vi "GenerateAnalogWaveformPiezoTraj - FeedPiezoGalvo - GalvoPrecision.vi"(8 "error in (no error)":errorcluster, 11 "SetupInfo_IN":T1={"ConfigParameters_Analog"={"JAI camera fps"=240.0, "Bi-Lateral Galvo xy scan range (V)"=0.7, "Bi-Lateral Galvo xy scan frequency (Hz)"=500, "AOM Blind percent (%)"=0.1, "AOM start blind percent (%) "=70.0, "ROI threshold"=1.0, "AO Sampling rate"=1000000.0}, "ConfigParameters_Digital"={"Steps per volume"=25.0, "Time per volume (s)"=0.4, "OG start layer"=15.0, "Objective Lin Rising Vel (micron/ms）"=1.0, "Image depth (micron)"=200.0, "OG latency (s)"=10.0, "OG repitation"=3.0, "OG end layer"=17.0, "Shock1 duration (s)"=0.001, "Shock2 duration (s)"=0.001, "Shock3 duration (s)"=0.01, "Shock4 duration (s)"=0.01, "Shock5 duration (s)"=0.1, "Shock duration_New"=[]}, "ConfigParameters_Other1"={"Frontal Galvo xy scan range (V)"=0.14, "Frontal Galvo xy scan frequency (Hz)"=500, "PFI 0 digital clock frequency"=500000.0, "Window size for layer index"=0.5, "sCMOS fps"=95.0}, "ConfigParameters_Others2"={"#Trials baseline"=6, "#Trials test"=6, "Time before acq. (s)"=360.0, "Time before test (s)"=600.0, "#Blocks acquisition"=5, "Inter-trial interval baseline (s)"=60.0, "#Trials per acquition block"=6, "Inter-block interval acquisition (s)"=360.0, "Inter-trial interval acquisition (s)"=20.0, "Flash latency (s)"=10.0, "Flash duration (s)"=3.2, "Response duration (s)"=10.0, "MaxTimeEventDetection (s)"=6, "StimType"=enum."Flash", "#MaxEvents"=6}, "ProcessParametersOut"={"stand Z vol Acquisition time (s)"=0.2631578947368421, "stand Z vol Backward time (s)"=0.13684210526315793, "Objective scan volt"=5.0, "Bi-lateral Galvo Z scan volt"=0.1800000180000018, "Frontal Galvo Z scan volt"=0.14940000509752818, "Objective step length (micron)"=8.0, "OG Z volet Linear Dec time (s)"=0.024, "OG Z vol Stim. steps time (s)"=0.031578947368421054, "OG Z vol Linear Acc time (s)"=0.112, "#Vol. of flash"=8, "#Vol. of shock"=1, "#Vol. bef flash"=25, "#Vol. aft flash"=17, "OG Z vol Linear Dec time (s)"=0.112, "OG Z vol time (s)"=0.39073684210526316, "Stack duration"=[0.001, 0.001, 0.01, 0.01, 0.1], "AOM stand. value size"=400000, "Plane indexing length"=0, "#Vol. blank"=0, "#Vol. blank before acq"=0, "#Vol. blank before test"=0, " #Inter-block interval acquisition (Ed-St Vol)"=0}, "WaveformParameters"={"stand Z vol Acquisition samp info"={"Fs"=1000000.0, "#s"=263158.0}, "stand Z vol Backward samp info"={"Fs"=1000000.0, "#s"=136842.0}, "OG Z vol Linear Acc samp info"={"Fs"=1000000.0, "#s"=112000.0}, "OG Z vol Stim. steps samp info"={"Fs"=1000000.0, "#s"=31579.0}, "OG Z volet Linear Dec samp info"={"Fs"=1000000.0, "#s"=24000.0}, "OG Z vol Linear Dec samp info"={"Fs"=1000000.0, "#s"=112000.0}, "OG Z vol samp info"={"Fs"=1000000.0, "#s"=390737.0}, "stand Z vol backforth samp info"={"Fs"=1000000.0, "#s"=400000.0}}, "AnalogWaveform"={"Bi-lateral Galvo Z stand waveform"={"t0"=timestamp(0 s since 1904-01-01), "dt"=1.0, "Y"=[]}, "Frontal Galvo Z stand waveform"={"t0"=timestamp(0 s since 1904-01-01), "dt"=1.0, "Y"=[]}, "Bi-lateral Galvo XY stand waveform"={"t0"=timestamp(0 s since 1904-01-01), "dt"=1.0, "Y"=[]}, "Frontal Galvo XY stand waveform"={"t0"=timestamp(0 s since 1904-01-01), "dt"=1.0, "Y"=[]}, "sCMOS stand waveform"={"t0"=timestamp(0 s since 1904-01-01), "dt"=1.0, "Y"=[]}, "Detection objective stand waveform"={"t0"=timestamp(0 s since 1904-01-01), "dt"=1.0, "Y"=[]}, "AOM stand waveform"={"t0"=timestamp(0 s since 1904-01-01), "dt"=1.0, "Y"=[]}, "PFI 0 clock stand waveform"={"t0"=timestamp(0 s since 1904-01-01), "dt"=1.0, "Y"=[]}, "Bi-lateral Galvo Z OG waveform"={"t0"=timestamp(0 s since 1904-01-01), "dt"=1.0, "Y"=[]}, "Bi-lateral Galvo XY OG waveform"={"t0"=timestamp(0 s since 1904-01-01), "dt"=1.0, "Y"=[]}, "Frontal Galvo Z OG waveform"={"t0"=timestamp(0 s since 1904-01-01), "dt"=1.0, "Y"=[]}, "Frontal Galvo XY OG waveform"={"t0"=timestamp(0 s since 1904-01-01), "dt"=1.0, "Y"=[]}, "sCMOS OG waveform"={"t0"=timestamp(0 s since 1904-01-01), "dt"=1.0, "Y"=[]}, "Detection objective OG waveform"={"t0"=timestamp(0 s since 1904-01-01), "dt"=1.0, "Y"=[]}, "AOM OG waveform"={"t0"=timestamp(0 s since 1904-01-01), "dt"=1.0, "Y"=[]}, "PFI 0 clock OG wavee"={"t0"=timestamp(0 s since 1904-01-01), "dt"=1.0, "Y"=[]}, "sCMOS blank waveform"={"t0"=timestamp(0 s since 1904-01-01), "dt"=1.0, "Y"=[]}, "All analog OG wave"=[], "All analog stand wave"=[], "All analog blank wave"=[], "BufferWaveform_Analog"=[], "Bi-lateral Galvo Z XY"={"t0"=timestamp(0 s since 1904-01-01), "dt"=1.0, "Y"=[]}, "Frontal Galvo Z XY"={"t0"=timestamp(0 s since 1904-01-01), "dt"=1.0, "Y"=[]}, "sCMOS Trigger XY"={"t0"=timestamp(0 s since 1904-01-01), "dt"=1.0, "Y"=[]}, "Detection objective XY"={"t0"=timestamp(0 s since 1904-01-01), "dt"=1.0, "Y"=[]}, "AOM XY"={"t0"=timestamp(0 s since 1904-01-01), "dt"=1.0, "Y"=[]}, "Analog_XY"=[]}, "DigitalWaveform"={"AllDigitalStandWave"=[], "AllDigialEvokedWave"=[], "AllDigialOGWave"=[], "AllDigitalPairWave_1"=[], "AllDigitalPairWave_2"=[], "AllDigitalPairWave_3"=[], "AllDigitalPairWave_4"=[], "AllDigitalPairWave_5"=[], "Plane Indexing"={"t0"=timestamp(0 s since 1904-01-01), "dt"=0.0, "Y"={"transitions"=[], "data"=[]}, "error"={"status"=FALSE, "code"=37421928, "source"=""}}, "Plane indexing P0.5 OG"={"t0"=timestamp(0 s since 1904-01-01), "dt"=0.0, "Y"={"transitions"=[], "data"=[]}, "error"={"status"=FALSE, "code"=37421928, "source"=""}}, "AllDigitalPairWaves"=[], "BufferWaveform_Digital"=[], "AllDigitalBlankWave"=[], "Digial_XY"=[]}, "PhysicalResource"={"PhysicalChannels_AI"="", "PhysicalChannels_AO"="", "PhysicalChannels_DO"="", "Task_AnalogOutput"="", "Task_DigitalOutput"="", "Task_AnalogInput"=""}, "ControlsRef"={"Mode_1"=refnum, "EventDetectionMode"=refnum, "Mode_2A"=refnum, "StimulationMode"=refnum, "Mode_2B"=refnum, "ErrorMeg"=refnum}} {"ConfigParameters_Other1"."Frontal Galvo xy scan frequency (Hz)" min=500 max=500; "ConfigParameters_Other1"."Frontal Galvo xy scan range (V)" min=0.0 max=1.5; "ConfigParameters_Analog"."AOM start blind percent (%)" min=10.0 max=90.0; "ConfigParameters_Analog"."AOM Blind percent (%)" min=0.1 max=100.0; "ConfigParameters_Analog"."Bi-Lateral Galvo xy scan frequency (Hz)" min=500 max=500; "ConfigParameters_Analog"."Bi-Lateral Galvo xy scan range (V)" min=0.0 max=1.5}) -> (0 "error out":errorcluster, 3 "SetupInfo_OUT":T1={"ConfigParameters_Analog"={"JAI camera fps"=240.0, "Bi-Lateral Galvo xy scan range (V)"=0.7, "Bi-Lateral Galvo xy scan frequency (Hz)"=500, "AOM Blind percent (%)"=0.1, "AOM start blind percent (%) "=70.0, "ROI threshold"=1.0, "AO Sampling rate"=1000000.0}, "ConfigParameters_Digital"={"Steps per volume"=25.0, "Time per volume (s)"=0.4, "OG start layer"=15.0, "Objective Lin Rising Vel (micron/ms）"=1.0, "Image depth (micron)"=200.0, "OG latency (s)"=10.0, "OG repitation"=3.0, "OG end layer"=17.0, "Shock1 duration (s)"=0.001, "Shock2 duration (s)"=0.001, "Shock3 duration (s)"=0.01, "Shock4 duration (s)"=0.01, "Shock5 duration (s)"=0.1, "Shock duration_New"=[]}, "ConfigParameters_Other1"={"Frontal Galvo xy scan range (V)"=0.14, "Frontal Galvo xy scan frequency (Hz)"=500, "PFI 0 digital clock frequency"=500000.0, "Window size for layer index"=0.5, "sCMOS fps"=95.0}, "ConfigParameters_Others2"={"#Trials baseline"=6, "#Trials test"=6, "Time before acq. (s)"=360.0, "Time before test (s)"=600.0, "#Blocks acquisition"=5, "Inter-trial interval baseline (s)"=60.0, "#Trials per acquition block"=6, "Inter-block interval acquisition (s)"=360.0, "Inter-trial interval acquisition (s)"=20.0, "Flash latency (s)"=10.0, "Flash duration (s)"=3.2, "Response duration (s)"=10.0, "MaxTimeEventDetection (s)"=6, "StimType"=enum."Flash", "#MaxEvents"=6}, "ProcessParametersOut"={"stand Z vol Acquisition time (s)"=0.2631578947368421, "stand Z vol Backward time (s)"=0.13684210526315793, "Objective scan volt"=5.0, "Bi-lateral Galvo Z scan volt"=0.1800000180000018, "Frontal Galvo Z scan volt"=0.14940000509752818, "Objective step length (micron)"=8.0, "OG Z volet Linear Dec time (s)"=0.024, "OG Z vol Stim. steps time (s)"=0.031578947368421054, "OG Z vol Linear Acc time (s)"=0.112, "#Vol. of flash"=8, "#Vol. of shock"=1, "#Vol. bef flash"=25, "#Vol. aft flash"=17, "OG Z vol Linear Dec time (s)"=0.112, "OG Z vol time (s)"=0.39073684210526316, "Stack duration"=[0.001, 0.001, 0.01, 0.01, 0.1], "AOM stand. value size"=400000, "Plane indexing length"=0, "#Vol. blank"=0, "#Vol. blank before acq"=0, "#Vol. blank before test"=0, " #Inter-block interval acquisition (Ed-St Vol)"=0}, "WaveformParameters"={"stand Z vol Acquisition samp info"={"Fs"=1000000.0, "#s"=263158.0}, "stand Z vol Backward samp info"={"Fs"=1000000.0, "#s"=136842.0}, "OG Z vol Linear Acc samp info"={"Fs"=1000000.0, "#s"=112000.0}, "OG Z vol Stim. steps samp info"={"Fs"=1000000.0, "#s"=31579.0}, "OG Z volet Linear Dec samp info"={"Fs"=1000000.0, "#s"=24000.0}, "OG Z vol Linear Dec samp info"={"Fs"=1000000.0, "#s"=112000.0}, "OG Z vol samp info"={"Fs"=1000000.0, "#s"=390737.0}, "stand Z vol backforth samp info"={"Fs"=1000000.0, "#s"=400000.0}}, "AnalogWaveform"={"Bi-lateral Galvo Z stand waveform"={"t0"=timestamp(0 s since 1904-01-01), "dt"=1.0, "Y"=[]}, "Frontal Galvo Z stand waveform"={"t0"=timestamp(0 s since 1904-01-01), "dt"=1.0, "Y"=[]}, "Bi-lateral Galvo XY stand waveform"={"t0"=timestamp(0 s since 1904-01-01), "dt"=1.0, "Y"=[]}, "Frontal Galvo XY stand waveform"={"t0"=timestamp(0 s since 1904-01-01), "dt"=1.0, "Y"=[]}, "sCMOS stand waveform"={"t0"=timestamp(0 s since 1904-01-01), "dt"=1.0, "Y"=[]}, "Detection objective stand waveform"={"t0"=timestamp(0 s since 1904-01-01), "dt"=1.0, "Y"=[]}, "AOM stand waveform"={"t0"=timestamp(0 s since 1904-01-01), "dt"=1.0, "Y"=[]}, "PFI 0 clock stand waveform"={"t0"=timestamp(0 s since 1904-01-01), "dt"=1.0, "Y"=[]}, "Bi-lateral Galvo Z OG waveform"={"t0"=timestamp(0 s since 1904-01-01), "dt"=1.0, "Y"=[]}, "Bi-lateral Galvo XY OG waveform"={"t0"=timestamp(0 s since 1904-01-01), "dt"=1.0, "Y"=[]}, "Frontal Galvo Z OG waveform"={"t0"=timestamp(0 s since 1904-01-01), "dt"=1.0, "Y"=[]}, "Frontal Galvo XY OG waveform"={"t0"=timestamp(0 s since 1904-01-01), "dt"=1.0, "Y"=[]}, "sCMOS OG waveform"={"t0"=timestamp(0 s since 1904-01-01), "dt"=1.0, "Y"=[]}, "Detection objective OG waveform"={"t0"=timestamp(0 s since 1904-01-01), "dt"=1.0, "Y"=[]}, "AOM OG waveform"={"t0"=timestamp(0 s since 1904-01-01), "dt"=1.0, "Y"=[]}, "PFI 0 clock OG wavee"={"t0"=timestamp(0 s since 1904-01-01), "dt"=1.0, "Y"=[]}, "sCMOS blank waveform"={"t0"=timestamp(0 s since 1904-01-01), "dt"=1.0, "Y"=[]}, "All analog OG wave"=[], "All analog stand wave"=[], "All analog blank wave"=[], "BufferWaveform_Analog"=[], "Bi-lateral Galvo Z XY"={"t0"=timestamp(0 s since 1904-01-01), "dt"=1.0, "Y"=[]}, "Frontal Galvo Z XY"={"t0"=timestamp(0 s since 1904-01-01), "dt"=1.0, "Y"=[]}, "sCMOS Trigger XY"={"t0"=timestamp(0 s since 1904-01-01), "dt"=1.0, "Y"=[]}, "Detection objective XY"={"t0"=timestamp(0 s since 1904-01-01), "dt"=1.0, "Y"=[]}, "AOM XY"={"t0"=timestamp(0 s since 1904-01-01), "dt"=1.0, "Y"=[]}, "Analog_XY"=[]}, "DigitalWaveform"={"AllDigitalStandWave"=[], "AllDigialEvokedWave"=[], "AllDigialOGWave"=[], "AllDigitalPairWave_1"=[], "AllDigitalPairWave_2"=[], "AllDigitalPairWave_3"=[], "AllDigitalPairWave_4"=[], "AllDigitalPairWave_5"=[], "Plane Indexing"={"t0"=timestamp(0 s since 1904-01-01), "dt"=0.0, "Y"={"transitions"=[], "data"=[]}, "error"={"status"=FALSE, "code"=37421928, "source"=""}}, "Plane indexing P0.5 OG"={"t0"=timestamp(0 s since 1904-01-01), "dt"=0.0, "Y"={"transitions"=[], "data"=[]}, "error"={"status"=FALSE, "code"=37421928, "source"=""}}, "AllDigitalPairWaves"=[], "BufferWaveform_Digital"=[], "AllDigitalBlankWave"=[], "Digial_XY"=[]}, "PhysicalResource"={"PhysicalChannels_AI"="", "PhysicalChannels_AO"="", "PhysicalChannels_DO"="", "Task_AnalogOutput"="", "Task_DigitalOutput"="", "Task_AnalogInput"=""}, "ControlsRef"={"Mode_1"=refnum, "EventDetectionMode"=refnum, "Mode_2A"=refnum, "StimulationMode"=refnum, "Mode_2B"=refnum, "ErrorMeg"=refnum}} {"ConfigParameters_Other1"."Frontal Galvo xy scan frequency (Hz)" min=500 max=500; "ConfigParameters_Other1"."Frontal Galvo xy scan range (V)" min=0.0 max=1.5; "ConfigParameters_Analog"."AOM start blind percent (%)" min=10.0 max=90.0; "ConfigParameters_Analog"."AOM Blind percent (%)" min=0.1 max=100.0; "ConfigParameters_Analog"."Bi-Lateral Galvo xy scan frequency (Hz)" min=500 max=500; "ConfigParameters_Analog"."Bi-Lateral Galvo xy scan range (V)" min=0.0 max=1.5})   [LabVIEW 2018]
uses:
  SetupInfo.ctl
  ConfigParameters_Analog.ctl
  ConfigParameters_Digital.ctl
  ConfigParameters_Others1.ctl
  ConfigParameters_Others2.ctl
  ProcessParametersOut.ctl
  WaveformParameters.ctl
  AnalogWaveform.ctl
  DigitalWaveform.ctl
  PhysicalResource.ctl
  ControlsRef.ctl
  <vilib>/Waveform/WDTOps.llb/WDT Append Waveforms DBL.vi
  <vilib>/measure/NI_MABase.lvlib
panel:
  out "x/y":waveform(dbl)(graph)
  in  "FileSamplingRate":dbl=1000.0
  in  "PiezoTrajectoryPath":path=path "D:/APP/LightSheetController_Ver8 obl/VISource/Waveform/piezo_In_Out.txt"
  out "AOM stand. value size":i32=400000
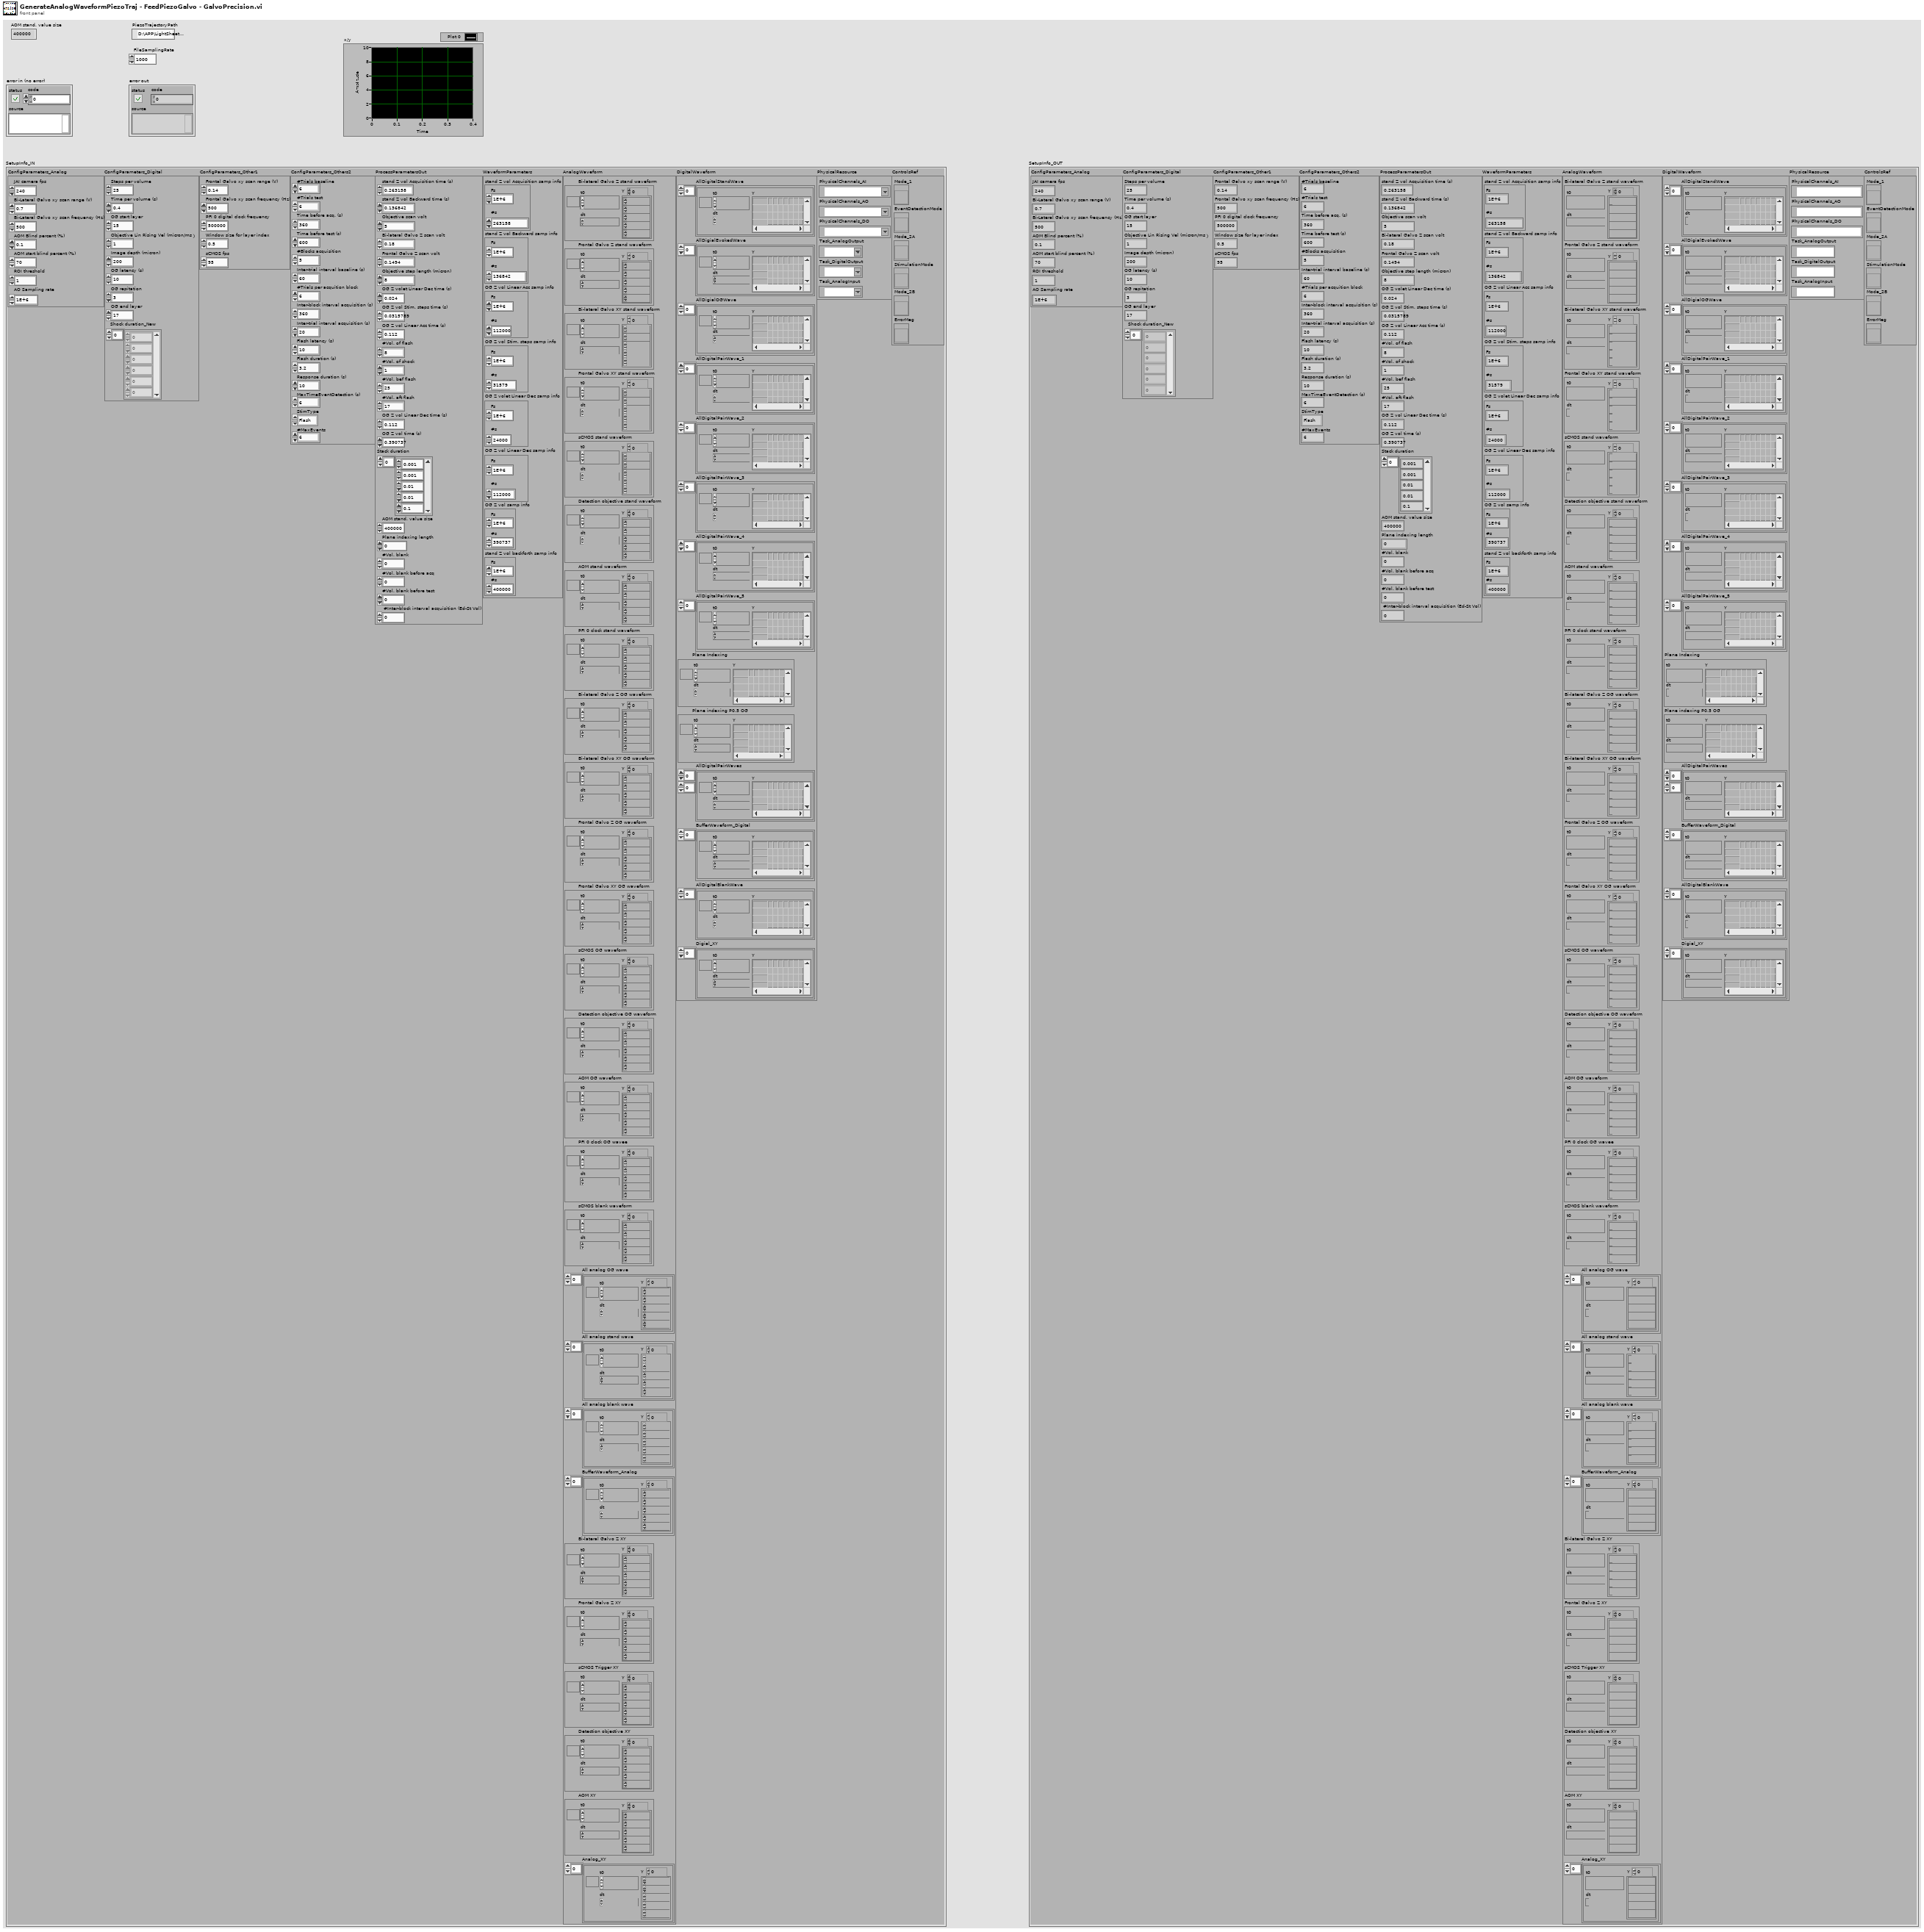
[diagram p1: front panel]
types:
  T1 = typedef "SetupInfo.ctl" = cluster{"ConfigParameters_Analog":T2, "ConfigParameters_Digital":T3, "ConfigParameters_Other1":T4, "ConfigParameters_Others2":T5, "ProcessParametersOut":T6, "WaveformParameters":T7, "AnalogWaveform":T8, "DigitalWaveform":T9, "PhysicalResource":T10, "ControlsRef":T11}
  T2 = typedef "ConfigParameters_Analog.ctl" = cluster{"JAI camera fps":dbl, "Bi-Lateral Galvo xy scan range (V)":dbl, "Bi-Lateral Galvo xy scan frequency (Hz)":i16, "AOM Blind percent (%)":dbl, "AOM start blind percent (%) ":dbl, "ROI threshold":dbl, "AO Sampling rate":dbl}
  T3 = typedef "ConfigParameters_Digital.ctl" = cluster{"Steps per volume":dbl, "Time per volume (s)":dbl, "OG start layer":dbl, "Objective Lin Rising Vel (micron/ms）":dbl, "Image depth (micron)":dbl, "OG latency (s)":dbl, "OG repitation":dbl, "OG end layer":dbl, "Shock1 duration (s)":dbl, "Shock2 duration (s)":dbl, "Shock3 duration (s)":dbl, "Shock4 duration (s)":dbl, "Shock5 duration (s)":dbl, "Shock duration_New":dbl[]}
  T4 = typedef "ConfigParameters_Others1.ctl" = cluster{"Frontal Galvo xy scan range (V)":dbl, "Frontal Galvo xy scan frequency (Hz)":i16, "PFI 0 digital clock frequency":dbl, "Window size for layer index":dbl, "sCMOS fps":dbl}
  T5 = typedef "ConfigParameters_Others2.ctl" = cluster{"#Trials baseline":i32, "#Trials test":i32, "Time before acq. (s)":dbl, "Time before test (s)":dbl, "#Blocks acquisition":i32, "Inter-trial interval baseline (s)":dbl, "#Trials per acquition block":i32, "Inter-block interval acquisition (s)":dbl, "Inter-trial interval acquisition (s)":dbl, "Flash latency (s)":dbl, "Flash duration (s)":dbl, "Response duration (s)":dbl, "MaxTimeEventDetection (s)":i32, "StimType":enum16{"Flash", "OG"}, "#MaxEvents":i32}
  T6 = typedef "ProcessParametersOut.ctl" = cluster{"stand Z vol Acquisition time (s)":dbl, "stand Z vol Backward time (s)":dbl, "Objective scan volt":dbl, "Bi-lateral Galvo Z scan volt":dbl, "Frontal Galvo Z scan volt":dbl, "Objective step length (micron)":dbl, "OG Z volet Linear Dec time (s)":dbl, "OG Z vol Stim. steps time (s)":dbl, "OG Z vol Linear Acc time (s)":dbl, "#Vol. of flash":i32, "#Vol. of shock":i32, "#Vol. bef flash":i32, "#Vol. aft flash":i32, "OG Z vol Linear Dec time (s)":dbl, "OG Z vol time (s)":dbl, "Stack duration":dbl[], "AOM stand. value size":i32, "Plane indexing length":i32, "#Vol. blank":i32, "#Vol. blank before acq":i32, "#Vol. blank before test":i32, " #Inter-block interval acquisition (Ed-St Vol)":i32}
  T7 = typedef "WaveformParameters.ctl" = cluster{"stand Z vol Acquisition samp info":cluster{"Fs":dbl, "#s":dbl}, "stand Z vol Backward samp info":cluster{"Fs":dbl, "#s":dbl}, "OG Z vol Linear Acc samp info":cluster{"Fs":dbl, "#s":dbl}, "OG Z vol Stim. steps samp info":cluster{"Fs":dbl, "#s":dbl}, "OG Z volet Linear Dec samp info":cluster{"Fs":dbl, "#s":dbl}, "OG Z vol Linear Dec samp info":cluster{"Fs":dbl, "#s":dbl}, "OG Z vol samp info":cluster{"Fs":dbl, "#s":dbl}, "stand Z vol backforth samp info":cluster{"Fs":dbl, "#s":dbl}}
  T8 = typedef "AnalogWaveform.ctl" = cluster{"Bi-lateral Galvo Z stand waveform":waveform(dbl), "Frontal Galvo Z stand waveform":waveform(dbl), "Bi-lateral Galvo XY stand waveform":waveform(dbl), "Frontal Galvo XY stand waveform":waveform(dbl), "sCMOS stand waveform":waveform(dbl), "Detection objective stand waveform":waveform(dbl), "AOM stand waveform":waveform(dbl), "PFI 0 clock stand waveform":waveform(dbl), "Bi-lateral Galvo Z OG waveform":waveform(dbl), "Bi-lateral Galvo XY OG waveform":waveform(dbl), "Frontal Galvo Z OG waveform":waveform(dbl), "Frontal Galvo XY OG waveform":waveform(dbl), "sCMOS OG waveform":waveform(dbl), "Detection objective OG waveform":waveform(dbl), "AOM OG waveform":waveform(dbl), "PFI 0 clock OG wavee":waveform(dbl), "sCMOS blank waveform":waveform(dbl), "All analog OG wave":waveform(dbl)[], "All analog stand wave":waveform(dbl)[], "All analog blank wave":waveform(dbl)[], "BufferWaveform_Analog":waveform(dbl)[], "Bi-lateral Galvo Z XY":waveform(dbl), "Frontal Galvo Z XY":waveform(dbl), "sCMOS Trigger XY":waveform(dbl), "Detection objective XY":waveform(dbl), "AOM XY":waveform(dbl), "Analog_XY":waveform(dbl)[]}
  T9 = typedef "DigitalWaveform.ctl" = cluster{"AllDigitalStandWave":digitalwaveform[], "AllDigialEvokedWave":digitalwaveform[], "AllDigialOGWave":digitalwaveform[], "AllDigitalPairWave_1":digitalwaveform[], "AllDigitalPairWave_2":digitalwaveform[], "AllDigitalPairWave_3":digitalwaveform[], "AllDigitalPairWave_4":digitalwaveform[], "AllDigitalPairWave_5":digitalwaveform[], "Plane Indexing":digitalwaveform, "Plane indexing P0.5 OG":digitalwaveform, "AllDigitalPairWaves":digitalwaveform[][], "BufferWaveform_Digital":digitalwaveform[], "AllDigitalBlankWave":digitalwaveform[], "Digial_XY":digitalwaveform[]}
  T10 = typedef "PhysicalResource.ctl" = cluster{"PhysicalChannels_AI":tag, "PhysicalChannels_AO":tag, "PhysicalChannels_DO":tag, "Task_AnalogOutput":refnum<k21>, "Task_DigitalOutput":refnum<k21>, "Task_AnalogInput":refnum<k21>}
  T11 = typedef "ControlsRef.ctl" = cluster{"Mode_1":refnum<vi>, "EventDetectionMode":refnum<vi>, "Mode_2A":refnum<vi>, "StimulationMode":refnum<vi>, "Mode_2B":refnum<vi>, "ErrorMeg":refnum<vi>}
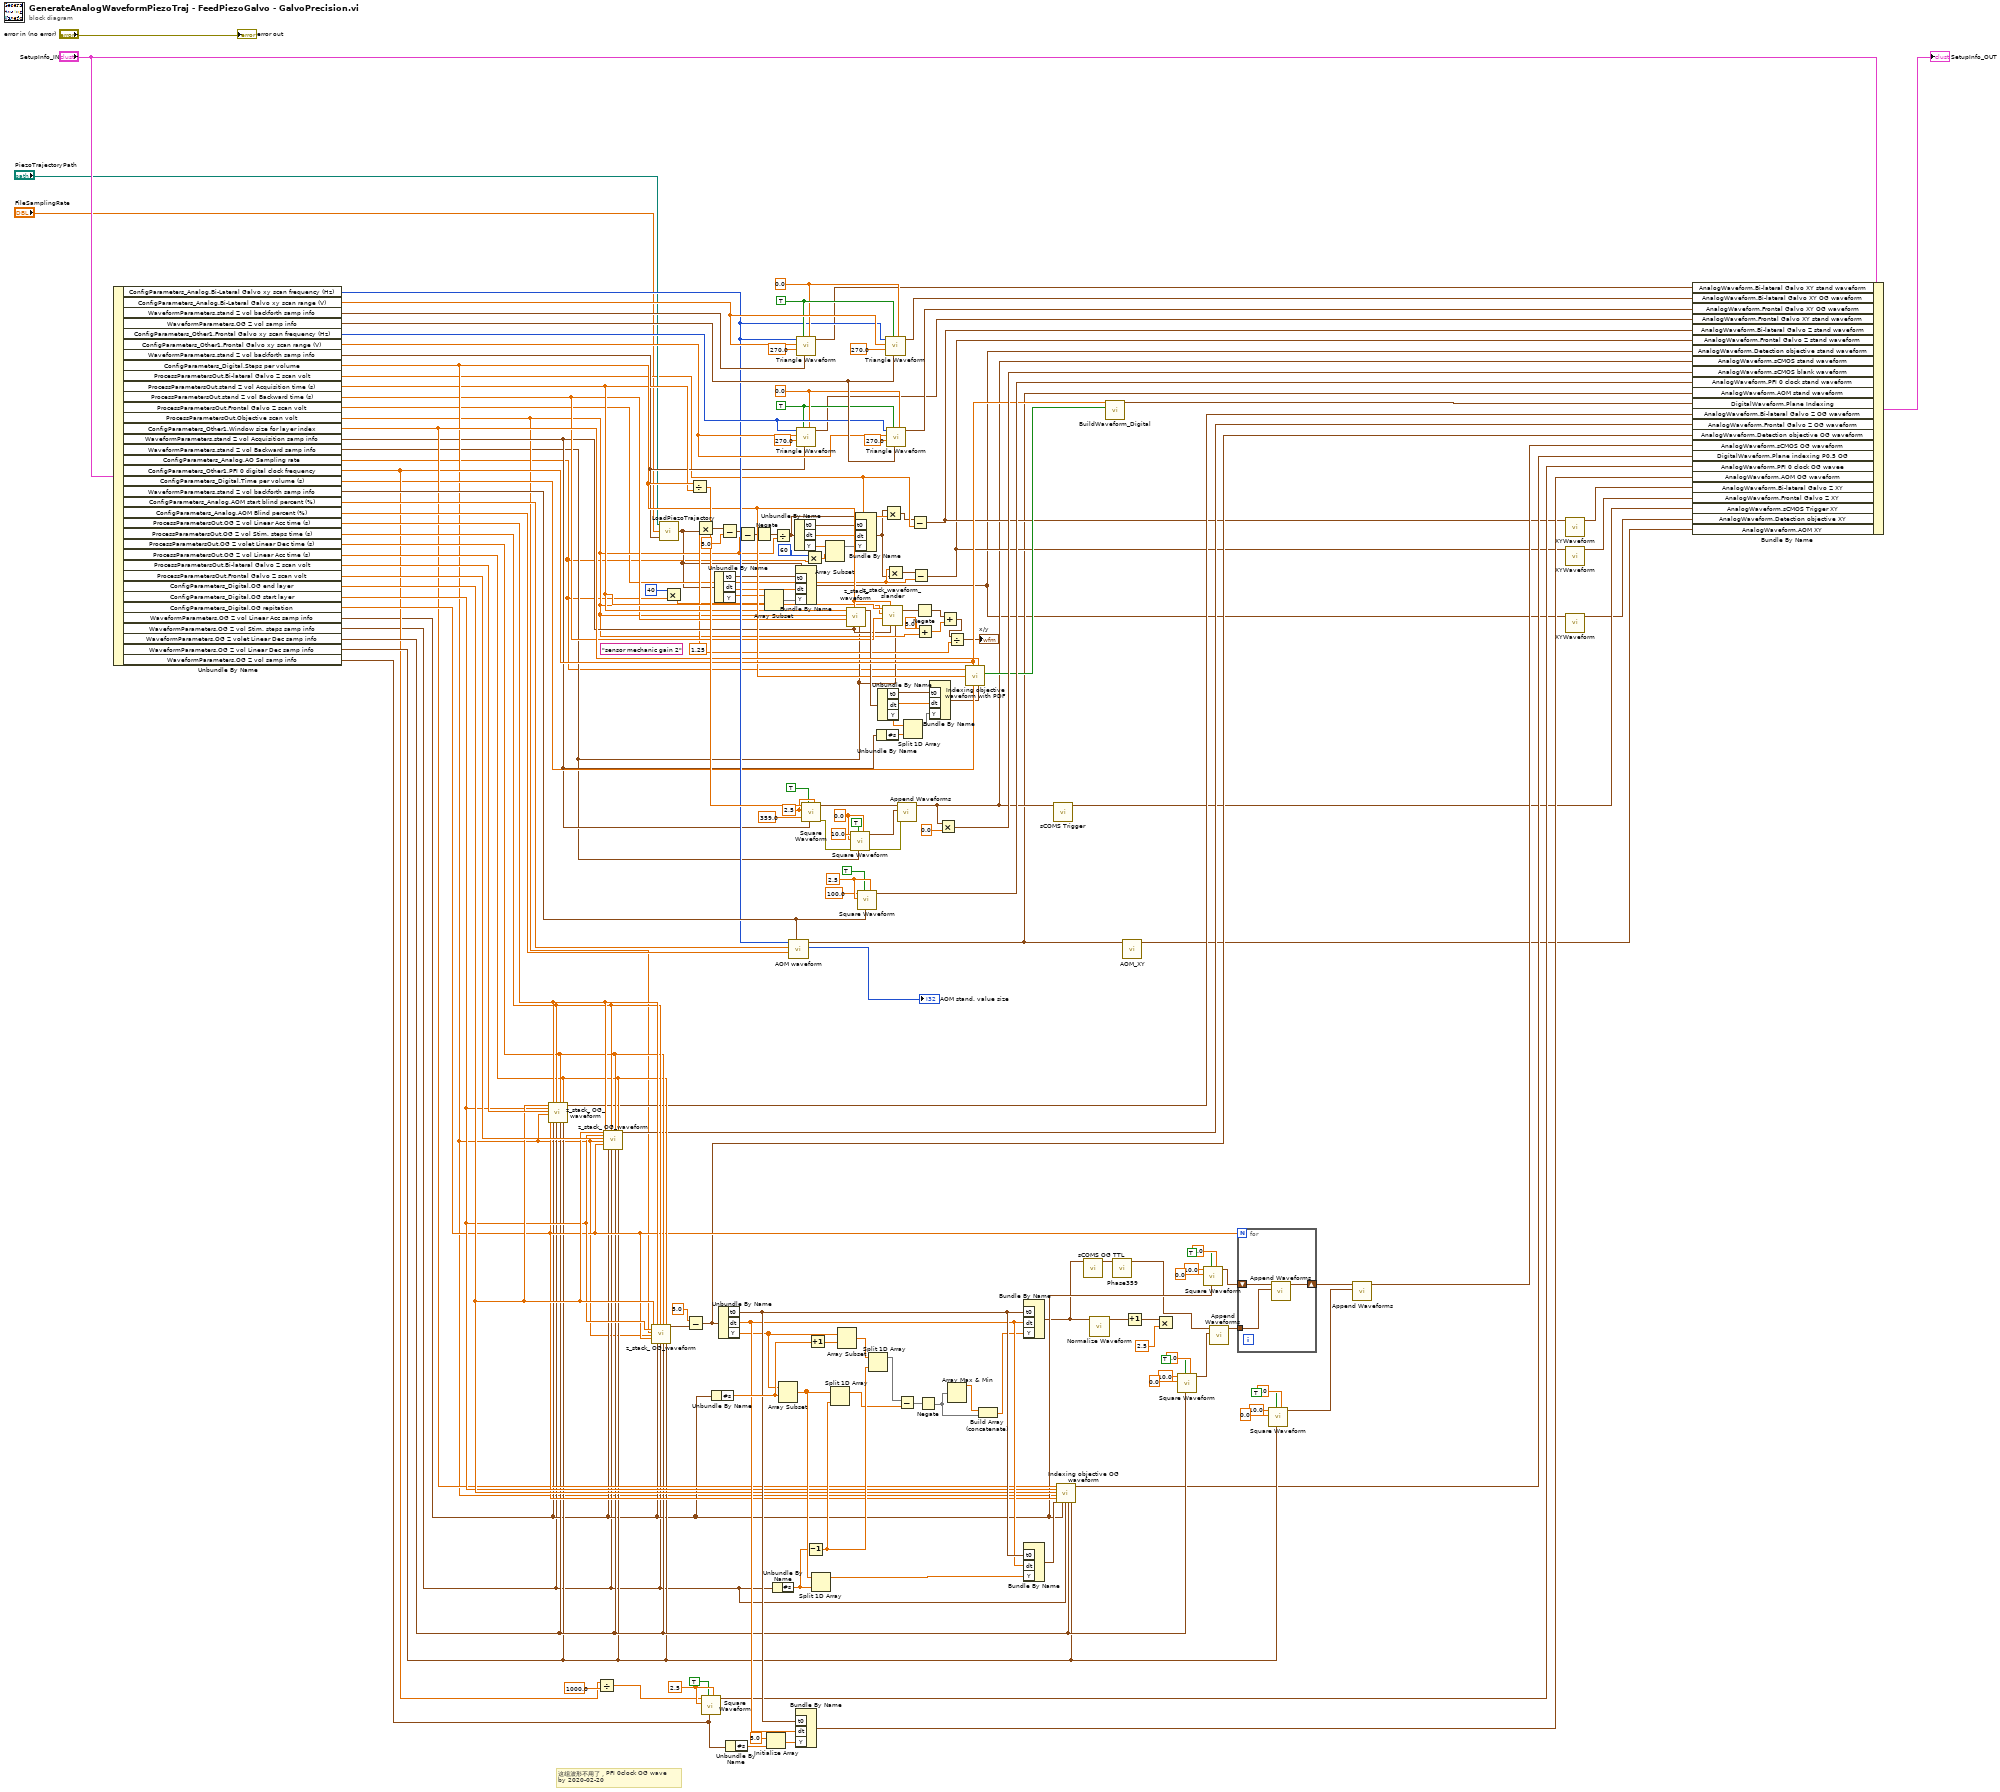
[diagram p0: block diagram]
diagram:
  (unwired) "sensor mechanic gain 2"
  w32 = 1.25
  w106 = 2.5
  w150 = 2.5 ("offset")
  w157 = 0.0 ("offset")
  w161 = 2.5 ("amplitude")
  w136 = TRUE ("reset signal")
  w144 = TRUE ("reset signal")
  w143 = 0.0 ("offset")
  w137 = 0.0 ("offset")
  # "这组波形不用了，PFI 0clock OG wave\nby 2020-02-20"
  n1 = Unbundle By Name("SetupInfo_IN") -> ("ConfigParameters_Analog.Bi-Lateral Galvo xy scan frequency (Hz)"=w133:i16, "ConfigParameters_Analog.Bi-Lateral Galvo xy scan range (V)"=w146:dbl, "WaveformParameters.stand Z vol backforth samp info"=w145:cluster{"Fs":dbl, "#s":dbl}, "WaveformParameters.OG Z vol samp info"=w141:cluster{"Fs":dbl, "#s":dbl}, "ConfigParameters_Other1.Frontal Galvo xy scan frequency (Hz)"=w140:i16, "ConfigParameters_Other1.Frontal Galvo xy scan range (V)"=w139:dbl, "WaveformParameters.stand Z vol backforth samp info"=w34:cluster{"Fs":dbl, "#s":dbl}, "ConfigParameters_Digital.Steps per volume"=w39:dbl, "ProcessParametersOut.Bi-lateral Galvo Z scan volt"=w24:dbl, "ProcessParametersOut.stand Z vol Acquisition time (s)"=w38:dbl, "ProcessParametersOut.stand Z vol Backward time (s)"=w37:dbl, "ProcessParametersOut.Frontal Galvo Z scan volt"=w22:dbl, "ProcessParametersOut.Objective scan volt"=w25:dbl, "ConfigParameters_Other1.Window size for layer index"=w90:dbl, "WaveformParameters.stand Z vol Acquisition samp info"=w36:cluster{"Fs":dbl, "#s":dbl}, "WaveformParameters.stand Z vol Backward samp info"=w20:cluster{"Fs":dbl, "#s":dbl}, "ConfigParameters_Analog.AO Sampling rate"=w3:dbl, "ConfigParameters_Other1.PFI 0 digital clock frequency"=w74:dbl, "ConfigParameters_Digital.Time per volume (s)"=w73:dbl, "WaveformParameters.stand Z vol backforth samp info"=w134:cluster{"Fs":dbl, "#s":dbl}, "ConfigParameters_Analog.AOM start blind percent (%)"=w132:dbl, "ConfigParameters_Analog.AOM Blind percent (%)"=w131:dbl, "ProcessParametersOut.OG Z vol Linear Acc time (s)"=w99:dbl, "ProcessParametersOut.OG Z vol Stim. steps time (s)"=w98:dbl, "ProcessParametersOut.OG Z volet Linear Dec time (s)"=w97:dbl, "ProcessParametersOut.OG Z vol Linear Acc time (s)"=w96:dbl, "ProcessParametersOut.Bi-lateral Galvo Z scan volt"=w95:dbl, "ProcessParametersOut.Frontal Galvo Z scan volt"=w94:dbl, "ConfigParameters_Digital.OG end layer"=w93:dbl, "ConfigParameters_Digital.OG start layer"=w92:dbl, "ConfigParameters_Digital.OG repitation"=w91:dbl, "WaveformParameters.OG Z vol Linear Acc samp info"=w56:cluster{"Fs":dbl, "#s":dbl}, "WaveformParameters.OG Z vol Stim. steps samp info"=w55:cluster{"Fs":dbl, "#s":dbl}, "WaveformParameters.OG Z volet Linear Dec samp info"=w89:cluster{"Fs":dbl, "#s":dbl}, "WaveformParameters.OG Z vol Linear Dec samp info"=w88:cluster{"Fs":dbl, "#s":dbl}, "WaveformParameters.OG Z vol samp info"=w87:cluster{"Fs":dbl, "#s":dbl})
  n2 = call "z_stack_ OG_waveform.vi"("OG end layer"=w93, "OG start layer"=w92, "SPECIFIC scan volt"=w95, "Steps per volume"=w39, "OG repitation"=w91, "Objective线性加速时间"=w99, "OG Z stack 线性加速 采样信息"=w56, "Objective 刺激steps 时间（s）"=w98, "OG Z stack 刺激steps 采样信息"=w55, "Objective volet 线性减速 时间（s）"=w97, "OG Z volet 线性减速 采样信息"=w89, "Objective线性减速时间"=w96, "OG Z stack 线性减速 采样信息"=w88) -> ("waveform out"=w77:waveform(dbl))  [unwired: 2 in, 4 out]
  n3 = Divide(x=w74, y=1000.0) -> (x/y=w80:dbl)
  n4 = call "z_stack_ OG_waveform.vi"("OG end layer"=w93, "OG start layer"=w92, "SPECIFIC scan volt"=w94, "Steps per volume"=w39, "OG repitation"=w91, "Objective线性加速时间"=w99, "OG Z stack 线性加速 采样信息"=w56, "Objective 刺激steps 时间（s）"=w98, "OG Z stack 刺激steps 采样信息"=w55, "Objective volet 线性减速 时间（s）"=w97, "OG Z volet 线性减速 采样信息"=w89, "Objective线性减速时间"=w96, "OG Z stack 线性减速 采样信息"=w88) -> ("waveform out"=w76:waveform(dbl))  [unwired: 2 in, 4 out]
  n5 = call "z_stack_ OG_waveform.vi"("OG end layer"=w93, "OG start layer"=w92, "SPECIFIC scan volt"=w25, "Steps per volume"=w39, "OG repitation"=w91, "Objective线性加速时间"=w99, "OG Z stack 线性加速 采样信息"=w56, "Objective 刺激steps 时间（s）"=w98, "OG Z stack 刺激steps 采样信息"=w55, "Objective volet 线性减速 时间（s）"=w97, "OG Z volet 线性减速 采样信息"=w89, "Objective线性减速时间"=w96, "OG Z stack 线性减速 采样信息"=w88) -> ("waveform out"=w69:waveform(dbl))  [unwired: 2 in, 4 out]
  n6 = call "LoadPiezoTrajactory.vi"("Z backforth 采样信息"=w34, "File Sampling Rate"="FileSamplingRate", "Path"="PiezoTrajectoryPath") -> ("output waveform"=w8:waveform(dbl))
  n7 = Multiply(x=40, y=w3) -> (x*y=w5:dbl)
  n8 = Subtract(x=5.0, y=w69) -> (x-y=w64:waveform(dbl))
  n9 = Divide(x=w39, y=w38) -> (x/y=w162:dbl)
  n10 = Multiply(x=w32, y=w8) -> (x*y=w31:waveform(dbl))
  n11 = call <vilib>:"Square Waveform.vi"("offset"=w106, "sampling info"=w87, "reset signal"=TRUE, "amplitude"=w106, "frequency"=w80) -> ("signal out"=w85:waveform(dbl))  [unwired: 5 in, 1 out]
  n12 = Unbundle By Name(w56) -> ("#s"=w107:dbl)
  n13 = Unbundle By Name(w8) -> ("t0"=w10:timestamp, "dt"=w9:dbl, "Y"=w6:dbl[])
  n14 = Unbundle By Name(w64) -> ("t0"=w102:timestamp, "dt"=w101:dbl, "Y"=w67:dbl[])
  n15 = Subtract(x=w31, y=5.0) -> (x-y=w30:waveform(dbl))
  n16 = Unbundle By Name(w87) -> ("#s"=w100:dbl)
  n17 = Subtract(x=w30, y=w25) -> (x-y=w27:waveform(dbl))
  n18 = Negate(x=w27) -> (-x=w26:waveform(dbl))
  n19 = Array Subset(array=w6, index=w5) -> (w7:dbl[])  [unwired: 1 in]
  n20 = Initialize Array(5.0 ("element"), w100) -> (w103:dbl[])
  n21 = Unbundle By Name(w55) -> ("#s"=w108:dbl)
  n22 = Divide(x=w26, y=w25) -> (x/y=w13:waveform(dbl))
  n23 = Array Subset(array=w67, index=w107) -> (w124:dbl[])  [unwired: 1 in]
  n24 = call "AOM waveform.vi"("z stack 往复采样信息"=w134, "AOM Blind percent (%)"=w131, "AOM start blind percent (%)"=w132, "Bi-Lateral Galvo xy scan frequency (Hz)"=w133) -> ("数值"=→"AOM stand. value size":i32, "Waveform"=w41:waveform(dbl))  [unwired: 6 in]
  n25 = Unbundle By Name(w13) -> ("t0"=w14:timestamp, "dt"=w17:dbl, "Y"=w15:dbl[])
  n26 = Bundle By Name(cluster=w8, "t0"=w10, "dt"=w9, "Y"=w7) -> (w11:waveform(dbl))
  n27 = Bundle By Name("t0"=w102, "dt"=w101, "Y"=w103) -> (w84:waveform(dbl))  [unwired: 1 in]
  n28 = call <vilib>:"Triangle Waveform.vi"("offset"=w143, "sampling info"=w145, "reset signal"=w144, "phase"=270.0, "amplitude"=w146, "frequency"=w133) -> ("signal out"=w82:waveform(dbl))  [unwired: 4 in, 1 out]
  n29 = call <vilib>:"Triangle Waveform.vi"("offset"=w137, "sampling info"=w34, "reset signal"=w136, "phase"=270.0, "amplitude"=w139, "frequency"=w140) -> ("signal out"=w135:waveform(dbl))  [unwired: 4 in, 1 out]
  n30 = call <vilib>:"Square Waveform.vi"("offset"=w161, "sampling info"=w36, "reset signal"=TRUE, "phase"=359.0, "amplitude"=w161, "frequency"=w162) -> ("error out"=w155:errorcluster, "signal out"=w153:waveform(dbl))  [unwired: 4 in]
  n31 = Multiply(x=60, y=w3) -> (x*y=w4:dbl)
  n32 = Decrement(x=w108) -> (x-1=w125:dbl)
  n33 = Increment(x=w107) -> (x+1=w126:dbl)
  n34 = Split 1D Array(array=w124, index=w108) -> (first subarray=w123:dbl[])  [unwired: 1 out]
  n35 = Array Subset(array=w15, index=w4) -> (w12:dbl[])  [unwired: 1 in]
  n36 = Split 1D Array(array=w124, index=w125) -> (first subarray=w60:dbl[])  [unwired: 1 out]
  n37 = Array Subset(array=w67, index=w126) -> (w66:dbl[])  [unwired: 1 in]
  n38 = call "z_stack_waveform.vi"("Z stack backward"=w20, "Z stack acquisition"=w36, "Steps per Volume"=w39, "Backward Time (s)"=w37, "SPECIFIC scan volt"=w25, "Aquisition Time (s)"=w38) -> ("WaveformOut"=w71:waveform(dbl))  [unwired: 5 in]
  n39 = call <vilib>:"Square Waveform.vi"("offset"=w157, "sampling info"=w20, "reset signal"=TRUE, "error in (no error)"=w155, "amplitude"=w157, "frequency"=10.0) -> ("error out"=w152:errorcluster, "signal out"=w154:waveform(dbl))  [unwired: 4 in]
  n40 = Bundle By Name(cluster=w13, "t0"=w14, "dt"=w17, "Y"=w12) -> (w16:waveform(dbl))
  n41 = call <vilib>:"Square Waveform.vi"("offset"=w150, "sampling info"=w134, "reset signal"=TRUE, "amplitude"=w150, "frequency"=100.0 ("amplitude")) -> ("signal out"=w129:waveform(dbl))  [unwired: 5 in, 1 out]
  n42 = Split 1D Array(array=w66, index=w125) -> (first subarray=w61:dbl[])  [unwired: 1 out]
  n43 = Unbundle By Name(w36) -> ("#s"=w164:dbl)
  n44 = Unbundle By Name(w71) -> ("t0"=w167:timestamp, "dt"=w166:dbl, "Y"=w165:dbl[])
  n45 = call "z_stack_waveform_slander.vi"("Z stack backward"=w20, "Z stack acquisition"=w36, "Steps per Volume"=w39, "Backward Time (s)"=w37, "SPECIFIC scan volt"=w25, "Aquisition Time (s)"=w38) -> ("WaveformOut"=w40:waveform(dbl))  [unwired: 5 in]
  n46 = Multiply(x=w16, y=w24) -> (x*y=w23:waveform(dbl))
  n47 = call <vilib>:"Triangle Waveform.vi"("offset"=w143, "sampling info"=w141, "reset signal"=w144, "phase"=270.0, "amplitude"=w146, "frequency"=w133) -> ("signal out"=w142:waveform(dbl))  [unwired: 4 in, 1 out]
  n48 = Multiply(x=w22, y=w16) -> (x*y=w21:waveform(dbl))
  n49 = call <vilib>:"Triangle Waveform.vi"("offset"=w137, "sampling info"=w141, "reset signal"=w136, "phase"=270.0, "amplitude"=w139, "frequency"=w140) -> ("signal out"=w138:waveform(dbl))  [unwired: 4 in, 1 out]
  n50 = call-poly <vilib>:"Append Waveforms.vi"("error in (no error)"=w152, "waveform B"=w154, "waveform A"=w153) -> ("waveform out"=w45:waveform(dbl))  [unwired: 7 in, 1 out]
  n51 = Subtract(x=w61, y=w60) -> (x-y=w58:dbl[])
  n52 = Split 1D Array(array=w165, index=w164) -> (first subarray=w163:dbl[])  [unwired: 1 out]
  n53 = Subtract(x=w23, y=w24) -> (x-y=w49:waveform(dbl))
  n54 = Subtract(x=w21, y=w22) -> (x-y=w47:waveform(dbl))
  n55 = Negate(x=w40) -> (-x=w169:waveform(dbl))
  n56 = Add(x=5.0, y=w25) -> (x+y=w168:dbl)
  n57 = Negate(x=w58) -> (-x=w65:dbl[])
  n58 = Bundle By Name("t0"=w167, "dt"=w166, "Y"=w163) -> (w72:waveform(dbl))  [unwired: 1 in]
  n59 = Multiply(x=w45, y=0.0) -> (x*y=w130:waveform(dbl))
  n60 = Add(x=w169, y=w168) -> (x+y=w35:waveform(dbl))
  n61 = Divide(x=w35, y=w32) -> (x/y=→"x/y":waveform(dbl))
  n62 = Array Max & Min(array=w65) -> (max value=w127:dbl)  [unwired: 3 out]
  n63 = call "Indexing objective waveform with PDF.vi"("AO sampling rate"=w3, "PFI0 digital clock frequency"=w74, "Steps per Volume"=w39, "Time per volume (s)"=w73, "Window size for layer index (ms)"=w90, "Steps Waveform"=w72) -> ("Plane Indexing data"=w79:bool[])  [unwired: 3 in, 1 out]
  n64 = Build Array (concatenate)(w127, w65) -> (w57:dbl[])
  n65 = Bundle By Name("t0"=w102, "dt"=w101, "Y"=w57) -> (w53:waveform(dbl))  [unwired: 1 in]
  n66 = Bundle By Name("t0"=w102, "dt"=w101, "Y"=w123) -> (w122:waveform(dbl))  [unwired: 1 in]
  n67 = call "sCOMS Trigger.vi"("In"=w45) -> ("Out"=w44:waveform(dbl))  [unwired: 10 in]
  n68 = call "Indexing objective OG waveform.vi"("Window size for layer index"=w90, "OG start layer"=w92, "OG end layer"=w93, "Steps per Volume"=w39, "OG repitation"=w91, "Waveform"=w122, "OG Z 线性加速 采样信息"=w56, "OG Z stack 刺激 steps 采样信息"=w55, "OG Z volet 线性减速 采样信息"=w89, "OG Z 线性减速 采样信息"=w88) -> ("Waveform_Digital"=w86:digitalwaveform)  [unwired: 9 in]
  n69 = call "sCOMS OG TTL.vi"("DataIn"=w53) -> ("Out"=w51:waveform(dbl))  [unwired: 10 in]
  n70 = call <vilib>:"Normalize Waveform.vi"("waveform in"=w53) -> ("normalized waveform"=w68:waveform(dbl))  [unwired: 7 in, 3 out]
  n71 = call "BuildWaveform_Digital.vi"("DigitalData"=w79, "SampleRate"=w74) -> ("DigitalWaveformOut"=w75:digitalwaveform)  [unwired: 9 in]
  n72 = call "Phase359.vi"("DataIn"=w51) -> ("DataOut"=w50:waveform(dbl))  [unwired: 10 in]
  n73 = call "AOM_XY.vi"("In"=w41) -> ("Out"=w42:waveform(dbl))  [unwired: 10 in]
  n74 = Increment(x=w68) -> (x+1=w70:waveform(dbl))
  n75 = Multiply(x=w70, y=2.5) -> ()  [unwired: 1 out]
  n76 = call <vilib>:"Square Waveform.vi"("offset"=0.0, "sampling info"=w89, "reset signal"=TRUE, "amplitude"=0.0, "frequency"=10.0) -> ("signal out"=w117:waveform(dbl))  [unwired: 5 in, 1 out]
  n77 = call <vilib>:"Square Waveform.vi"("offset"=0.0, "sampling info"=w56, "reset signal"=TRUE, "amplitude"=0.0, "frequency"=10.0) -> ("signal out"=w63:waveform(dbl))  [unwired: 5 in, 1 out]
  n78 = call-poly <vilib>:"Append Waveforms.vi"("waveform B"=w117, "waveform A"=w50) -> ("waveform out"=w62:waveform(dbl))  [unwired: 8 in, 1 out]
  n79 = for {
    N: w91 -> [_]
    tunnel: w62 -> [w178]
    shift-right: [w176] -> w54
    shift-left: w63 -> [w177]
    n80 = call-poly <vilib>:"Append Waveforms.vi"("waveform B"=w178, "waveform A"=w177) -> ("waveform out"=w176:waveform(dbl))  [unwired: 8 in, 1 out]
  }
  n81 = call <vilib>:"Square Waveform.vi"("offset"=0.0, "sampling info"=w88, "reset signal"=TRUE, "amplitude"=0.0, "frequency"=10.0) -> ("signal out"=w59:waveform(dbl))  [unwired: 5 in, 1 out]
  n82 = call-poly <vilib>:"Append Waveforms.vi"("waveform B"=w59, "waveform A"=w54) -> ("waveform out"=w52:waveform(dbl))  [unwired: 8 in, 1 out]
  n83 = call "XYWaveform.vi"("XYWaveformIN"=w49) -> ("XYWaveformOut"=w48:waveform(dbl))  [unwired: 10 in]
  n84 = call "XYWaveform.vi"("XYWaveformIN"=w47) -> ("XYWaveformOut"=w46:waveform(dbl))  [unwired: 10 in]
  n85 = call "XYWaveform.vi"("XYWaveformIN"=w11) -> ("XYWaveformOut"=w43:waveform(dbl))  [unwired: 10 in]
  n86 = Bundle By Name(cluster="SetupInfo_IN", "AnalogWaveform.Bi-lateral Galvo XY stand waveform"=w82, "AnalogWaveform.Bi-lateral Galvo XY OG waveform"=w142, "AnalogWaveform.Frontal Galvo XY OG waveform"=w138, "AnalogWaveform.Frontal Galvo XY stand waveform"=w135, "AnalogWaveform.Bi-lateral Galvo Z stand waveform"=w49, "AnalogWaveform.Frontal Galvo Z stand waveform"=w47, "AnalogWaveform.Detection objective stand waveform"=w11, "AnalogWaveform.sCMOS stand waveform"=w45, "AnalogWaveform.sCMOS blank waveform"=w130, "AnalogWaveform.PFI 0 clock stand waveform"=w129, "AnalogWaveform.AOM stand waveform"=w41, "DigitalWaveform.Plane Indexing"=w75, "AnalogWaveform.Bi-lateral Galvo Z OG waveform"=w77, "AnalogWaveform.Frontal Galvo Z OG waveform"=w76, "AnalogWaveform.Detection objective OG waveform"=w64, "AnalogWaveform.sCMOS OG waveform"=w52, "DigitalWaveform.Plane indexing P0.5 OG"=w86, "AnalogWaveform.PFI 0 clock OG wavee"=w85, "AnalogWaveform.AOM OG waveform"=w84, "AnalogWaveform.Bi-lateral Galvo Z XY"=w48, "AnalogWaveform.Frontal Galvo Z XY"=w46, "AnalogWaveform.sCMOS Trigger XY"=w44, "AnalogWaveform.Detection objective XY"=w43, "AnalogWaveform.AOM XY"=w42) -> (→"SetupInfo_OUT":T1)
  "error out" <- "error in (no error)"
